vi "get_offset_POSs.vi"(8 "error in (no error)":errorcluster caption="错误输入（无错误）", 11 "MotorSystem 输入":refnum<class "MotorSystem.lvclass">) -> (0 "error out":errorcluster caption="错误输出", 1 "pos without offset":dbl[](array[numeric]), 2 "pos with offset":dbl[](array[numeric]), 3 "MotorSystem 输出":refnum<class "MotorSystem.lvclass">)   [LabVIEW 2016, in "MotionControl_UFO_3DOF.lvlib" / "MotorSystem.lvclass"]
uses:
  <userlib>/MotionControl_UFO_3DOF/MotorSystem/MotorSystem.lvclass
  <userlib>/MotionControl_UFO_3DOF/MotorSystem/MotorSystem.lvclass/MotorSystem.ctl
  <userlib>/MotionControl_UFO_3DOF/OneMotion/OneMotion.lvclass
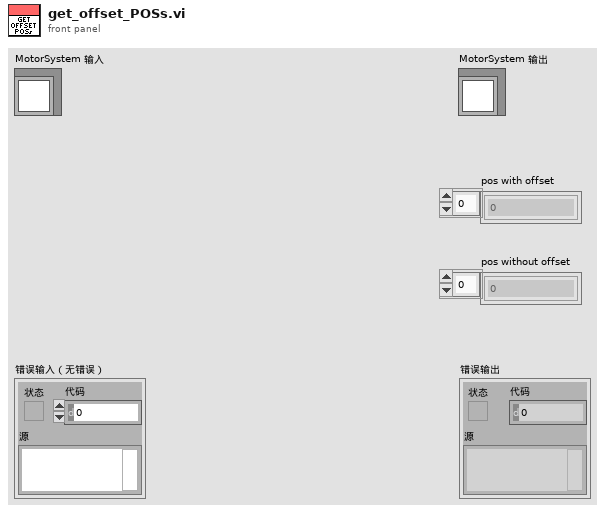
[diagram p1: front panel]
types:
  T1 = typedef "MotionControl_UFO_3DOF.lvlib/MotorSystem.lvclass/MotionCluster.ctl" = cluster{"OneMotion.lvclass":refnum<class "OneMotion.lvclass">, "connected?":bool, "default enabled?":bool, "enabled?":bool}
  T2 = typedef "MotionControl_UFO_3DOF.lvlib/OneMotion.lvclass/unit mode.ctl" = enum16{"motor (pulse)", "linear (mm) or radial (degree)"}
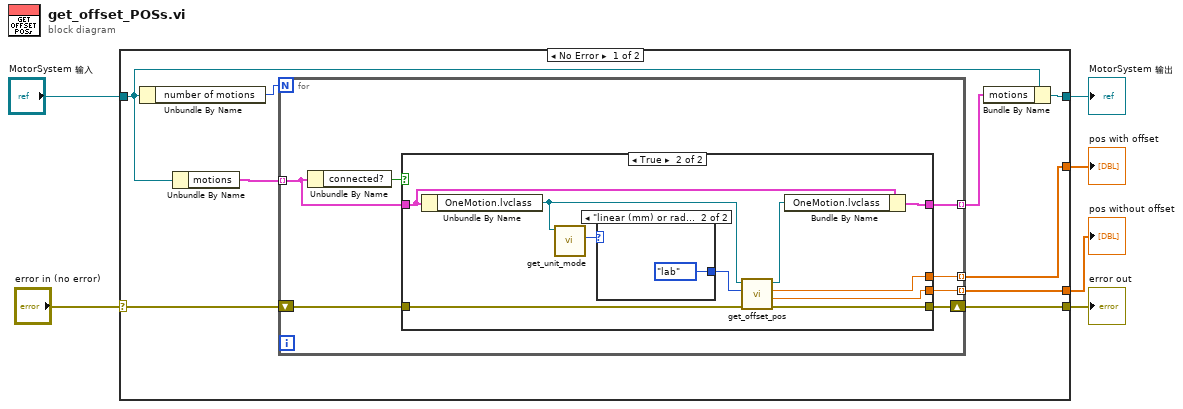
[diagram p0: block diagram]
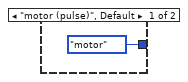
[diagram p3: hidden frame]
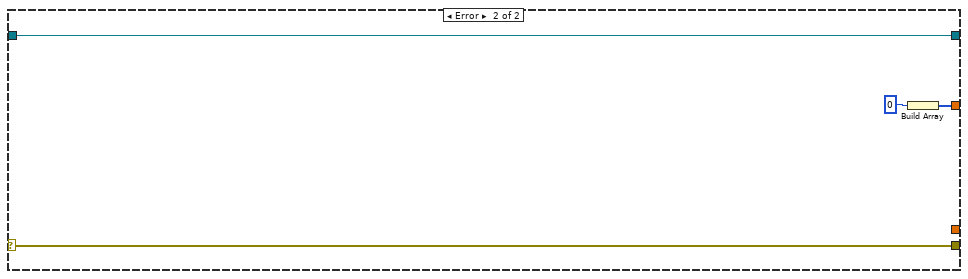
[diagram p4: hidden frame]
diagram:
  n1 = case shown="No Error" "error in (no error)" {
    selector: "error in (no error)" -> [w12 w40]
    tunnel: [w11 w40] -> w5
    tunnel: [w8 w39] -> w3
    tunnel: "MotorSystem 输入" -> [w10 w39]
    tunnel: [w13 w37] -> w2
    tunnel: [w7 _] -> w1
    frame No Error {
      n2 = Unbundle By Name(w10) -> ("number of motions"=w15:i32)
      n3 = Unbundle By Name(w10) -> ("motions"=w14:T1[])
      n4 = for {
        N: w15 -> [_]
        tunnel: w14 -> [w17] mode=indexing
        tunnel: [w20] -> w13 mode=indexing
        shift-right: [w21] -> w11
        shift-left: w12 -> [w22]
        tunnel: [w19] -> w9 mode=indexing
        tunnel: [w18] -> w7 mode=indexing
        n5 = Unbundle By Name(w17) -> ("connected?"=w16:bool)
        n6 = case shown="True" w16 {
          tunnel: w22 -> [w23 w34]
          tunnel: [w23 w33] -> w21
          tunnel: [_ w32] -> w20
          tunnel: w17 -> [w24 w31]
          tunnel: [w24 w29] -> w19
          tunnel: [_ w25] -> w18
          frame False {
          }
          frame True {
            n7 = Unbundle By Name(w31) -> ("OneMotion.lvclass"=w28:refnum<class "OneMotion.lvclass">)
            n8 = call-dynamic "get_unit_mode.vi"("OneMotion输入"=w28) -> ("unit mode"=w27:T2)  [unwired: 8 in, 2 out]
            n9 = case shown="\"linear (mm) or radial (degree)\"" w27 {
              tunnel: [enum16{"lab", "motor"}."motor" ("lab or motor") enum16{"lab", "motor"}."lab" ("lab or motor")] -> w26
              frame "motor (pulse)", Default {
              }
              frame "linear (mm) or radial (degree)" {
              }
            }
            n10 = call <userlib>:"get_offset_pos.vi"("error in (no error)"=w34, "lab or motor"=w26, "OneMotion 输入"=w28) -> ("error out"=w33:errorcluster, "pos without offset"=w25:dbl, "pos with offset"=w32:dbl, "OneMotion 输出"=w30:refnum<class "OneMotion.lvclass">)  [unwired: 5 in]
            n11 = Bundle By Name(cluster=w31, "OneMotion.lvclass"=w30) -> (w29:T1)
          }
        }
      }
      n12 = Bundle By Name(cluster=w10, "motions"=w9) -> (w8:refnum<class "MotorSystem.lvclass">)
    }
    frame Error {
      n13 = Build Array(0) -> (w37:i32[])
    }
  }
  "error out" <- w5
  "MotorSystem 输出" <- w3
  "pos with offset" <- w2
  "pos without offset" <- w1
